vi "min-max-y-cursors.vi"(0 "XYGraph in":refnum<vi>, 1 "GRAPH EXPERIMENTAL DATA ref":refnum<vi>) -> (2 "minY":dbl, 3 "maxY":dbl, 4 "minX":dbl, 5 "maxX":dbl)   [LabVIEW 2015]
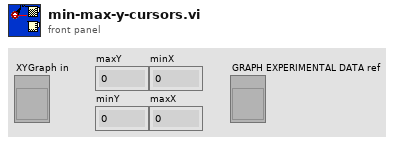
[diagram p1: front panel]
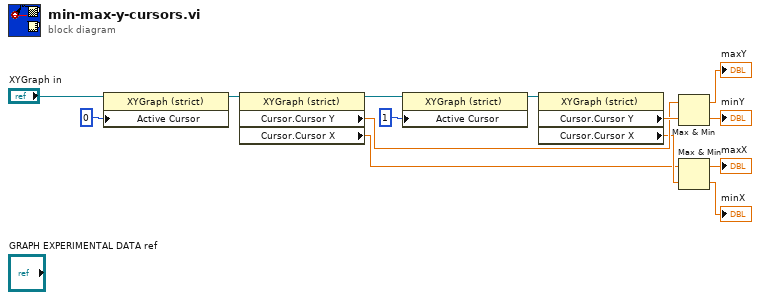
[diagram p0: block diagram]
diagram:
  n1 = property class="XYGraph (strict)"(reference="XYGraph in", "Active Cursor"=u32 0) -> (reference out=w5:refnum<vi>)  [unwired: 1 in, 1 out]
  n2 = property class="XYGraph (strict)"(reference=w5) -> (reference out=w6:refnum<vi>, "Cursor.Cursor Y"=w11:dbl, "Cursor.Cursor X"=w3:dbl)  [unwired: 1 in, 1 out]
  n3 = property class="XYGraph (strict)"(reference=w6, "Active Cursor"=u32 1) -> (reference out=w7:refnum<vi>)  [unwired: 1 in, 1 out]
  n4 = property class="XYGraph (strict)"(reference=w7) -> ("Cursor.Cursor Y"=w12:dbl, "Cursor.Cursor X"=w4:dbl)  [unwired: 1 in, 2 out]
  n5 = Max & Min(x=w11, y=w12) -> (max(x,y)=→"maxY":dbl, min(x,y)=→"minY":dbl)
  n6 = Max & Min(x=w3, y=w4) -> (max(x,y)=→"maxX":dbl, min(x,y)=→"minX":dbl)
